vi "CompressBuild.vi"(4 "LocalCompiledDir":path, 6 "DevMode":bool, 8 "error in":errorcluster, 11 "RasPi Compiler in":refnum<class "RasPi Compiler.lvclass">) -> (0 "error out":errorcluster, 3 "RasPi Compiler out":refnum<class "RasPi Compiler.lvclass">)   [LabVIEW 2014, in "Raspberry Pi Compatible Compiler for LabVIEW.lvlib" / "RasPi Compiler.lvclass"]
uses:
  RasPi Compiler.lvclass
  RasPi Compiler.lvclass/RasPi Compiler.ctl
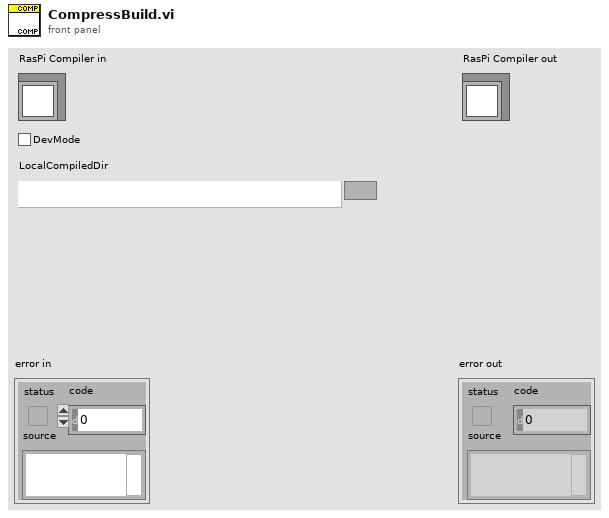
[diagram p1: front panel]
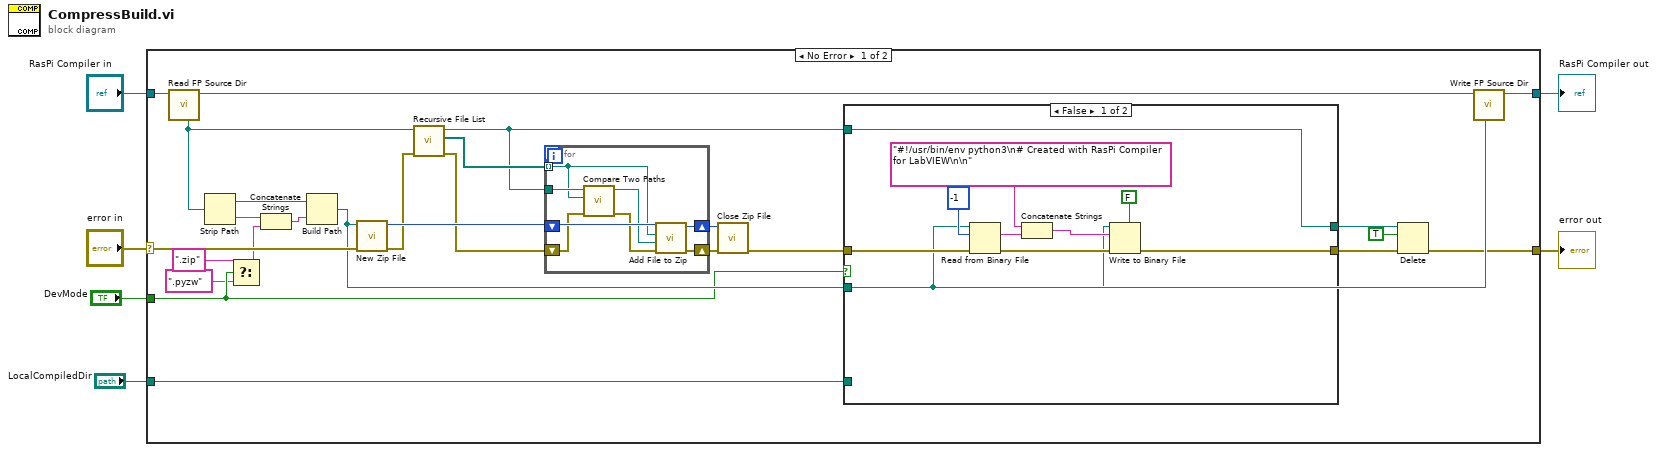
[diagram p0: block diagram]
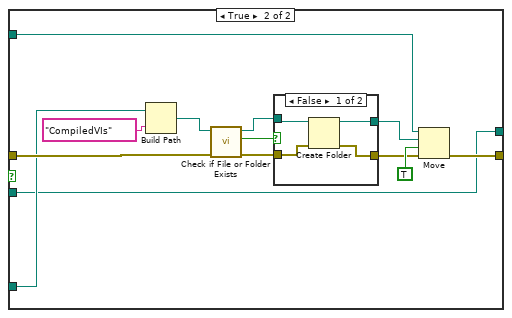
[diagram p2: hidden frame]
diagram:
  n1 = case shown="No Error" "error in" {
    selector: "error in" -> [w32 w70]
    tunnel: [w8 w70] -> w5
    tunnel: [w18 w69] -> w3
    tunnel: "RasPi Compiler in" -> [w30 w69]
    tunnel: "DevMode" -> [w16 _]
    tunnel: "LocalCompiledDir" -> [w12 _]
    frame No Error {
      n2 = call "Read FP Source Dir.vi"("RasPi Compiler in"=w30) -> ("RasPi Compiler out"=w19:refnum<class "RasPi Compiler.lvclass">, "FP Source Dir"=w23:path)  [unwired: 7 in]
      n3 = Strip Path(path=w23) -> (stripped path=w27:path, name=w29:string)
      n4 = Select(t=".zip" ("string"), s=w16, f=".pyzw" ("string")) -> (s? t:f=w13:string)
      n5 = Concatenate Strings(w29, w13) -> (w28:string)
      n6 = Build Path(base path=w27, name or relative path=w28) -> (appended path=w17:path)
      n7 = call <vilib>:"New Zip File.vi"("error in (no error)"=w32, "target"=w17) -> ("error out"=w22:errorcluster, "zip file out"=w31:i64)  [unwired: 3 in, 1 out]
      n8 = call <vilib>:"Recursive File List.vi"("error in (no error)"=w22, "Folder Path"=w23) -> ("error out"=w21:errorcluster, "All Files in Dir"=w20:path[], "dup Folder Path"=w11:path)  [unwired: 5 in, 2 out]
      n9 = for {
        shift-right: [w66] -> w25
        shift-left: w31 -> [w68]
        shift-right: [w67] -> w26
        shift-left: w21 -> [w65]
        tunnel: w11 -> [w62]
        tunnel: w20 -> [w61] mode=indexing
        n10 = call <vilib>:"Compare Two Paths.vi"("error in (no error)"=w65, "Path 2"=w61, "Path 1"=w62) -> ("error out"=w64:errorcluster, "Relative Path from 1 to 2"=w63:path)  [unwired: 5 in, 2 out]
        n11 = call <vilib>:"Add File to Zip.vi"("error in (no error)"=w64, "destination path in zip"=w63, "source file path"=w61, "zip file in"=w68) -> ("error out"=w67:errorcluster, "zip file out"=w66:i64)  [unwired: 6 in]
      }
      n12 = call <vilib>:"Close Zip File.vi"("error in (no error)"=w26, "zip file in"=w25) -> ("error out"=w10:errorcluster)  [unwired: 5 in]
      n13 = case shown="False" w16 {
        tunnel: w10 -> [w42 w49]
        tunnel: [w35 w54] -> w9
        tunnel: w17 -> [w34 w43]
        tunnel: w12 -> [_ w47]
        tunnel: [w33 w43] -> w7
        tunnel: w11 -> [w33 w44]
        frame False {
          n14 = Read from Binary File(8:w42, 10:-1 ("count (1)"), 11:w34) -> (0:w38:errorcluster, 2:w40:string)  [unwired: 3 in, 2 out]
          n15 = Concatenate Strings("#!/usr/bin/env python3\n# Created with RasPi Compiler for LabVIEW\n\n", w40) -> (w37:string)
          n16 = Write to Binary File(file (use dialog)=w34, data=w37, error in=w38, 5:FALSE ("prepend array or string size? (T)")) -> (error out=w35:errorcluster)  [unwired: 2 in, 2 out]
        }
        frame True {
          n17 = Build Path(base path=w47, name or relative path="CompiledVIs") -> (appended path=w51:path)
          n18 = call <vilib>:"Check if File or Folder Exists.vi"("error in (no error)"=w49, "path"=w51) -> ("error out"=w52:errorcluster, "file or folder exists?"=w50:bool)  [unwired: 7 in, 1 out]
          n19 = case shown="False" w50 {
            tunnel: w51 -> [w58 w60]
            tunnel: [w57 w60] -> w45
            tunnel: w52 -> [w56 w59]
            tunnel: [w55 w59] -> w48
            frame False {
              n20 = Create Folder(path (use dialog)=w58, error in=w56) -> (created path=w57:path, error out=w55:errorcluster)  [unwired: 1 in, 1 out]
            }
            frame True {
            }
          }
          n21 = Move(source path=w44, error in=w48, 9:TRUE ("overwrite (F)"), 10:w45) -> (error out=w54:errorcluster)  [unwired: 1 in, 2 out]
        }
      }
      n22 = Delete(path (use dialog)=w7, entire hierarchy (F)=TRUE, error in=w9) -> (error out=w8:errorcluster)  [unwired: 2 in, 2 out]
      n23 = call "Write FP Source Dir.vi"("FP Source Dir"=w17, "RasPi Compiler in"=w19) -> ("RasPi Compiler out"=w18:refnum<class "RasPi Compiler.lvclass">)  [unwired: 7 in]
    }
    frame Error {
    }
  }
  "error out" <- w5
  "RasPi Compiler out" <- w3
